vi "Steering Setpoint.vi"(1 "feildCentric":bool, 2 "rotation":dbl, 3 "joystickRight(x,y)":cluster{"X":dbl, "Y":dbl}, 4 "joystickLeft(x,y)":cluster{"X":dbl, "Y":dbl}) -> (0 "steerSetpoint":dbl[](array[numeric]))   [LabVIEW 2019]
panel:
  in  "steeringStay":dbl[](array[numeric])=[0.0]
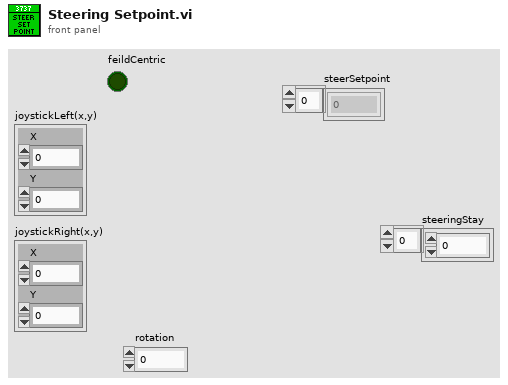
[diagram p1: front panel]
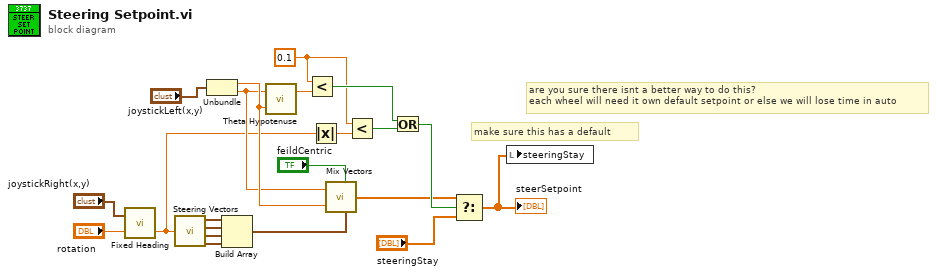
[diagram p0: block diagram]
diagram:
  w5 = 0.1
  # "are you sure there isnt a better way to do this?\neach wheel will need it own default setpoint or else we will lose time in auto"
  # "make sure this has a default"
  n1 = call "Fixed Heading.vi"("inputRotation"="rotation", "joystickHeading(x,y)"="joystickRight(x,y)") -> ("outputRotation"=w1:dbl)  [unwired: 1 in]
  n2 = call "Steering Vectors.vi"("rotation"=w1) -> ("BL Vector"=w18:cluster{dbl, dbl}, "BR Vector"=w19:cluster{dbl, dbl}, "FR Vector"=w20:cluster{dbl, dbl}, "FL Vector"=w21:cluster{dbl, dbl})  [unwired: 2 in]
  n3 = Unbundle("joystickLeft(x,y)") -> ("X"=w9:dbl, "Y"=w8:dbl)
  n4 = Build Array(w18, w19, w20, w21) -> (w17:cluster{dbl, dbl}[])
  n5 = call "Theta Hypotenuse.vi"("x value"=w9, "y value"=w8) -> ("Hypotenuse"=w16:dbl)  [unwired: 1 out]
  n6 = Less?(x=w5, y=w16) -> (x < y?=w13:bool)
  n7 = Absolute Value(x=w1) -> (abs(x)=w4:dbl)
  n8 = call "Mix Vectors.vi"("inputVectors"=w17, "feildCentric"="feildCentric", "x value"=w9, "y value"=w8) -> ("finalVectors"=w3:dbl[])  [unwired: 2 in]
  n9 = Less?(x=w5, y=w4) -> (x < y?=w6:bool)
  n10 = Or(x=w13, y=w6) -> (x .or. y?=w14:bool)
  n11 = Select(t=w3, s=w14, f="steeringStay") -> (s? t:f=w2:dbl[])
  "steerSetpoint" <- w2
  n12 = local write "steeringStay"(w2) -> ()
